vi "即时帮助.vi"() -> ()   [LabVIEW 2020]
panel:
  in  "确认":bool
  out "帮助信息":T1
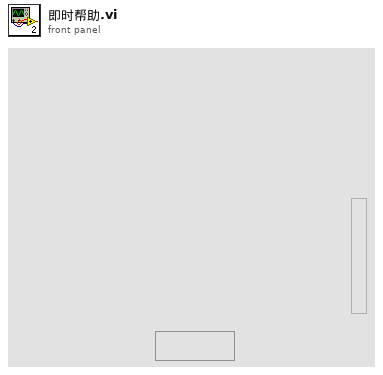
[diagram p1: front panel]
types:
  T1 = cluster{"名称":string, "图片":picture, "关键字":string, "程序文本":string}
  T2 = cluster{"名称":string, "关键字":string, "程序文本":string}
  T3 = typedef "imagedata.ctl" = cluster{"image type":i32, "image depth":i32, "image":u8[], "mask":u8[], "colors":u32[], "Rectangle":cluster{"left":i16, "top":i16, "right":i16, "bottom":i16}}
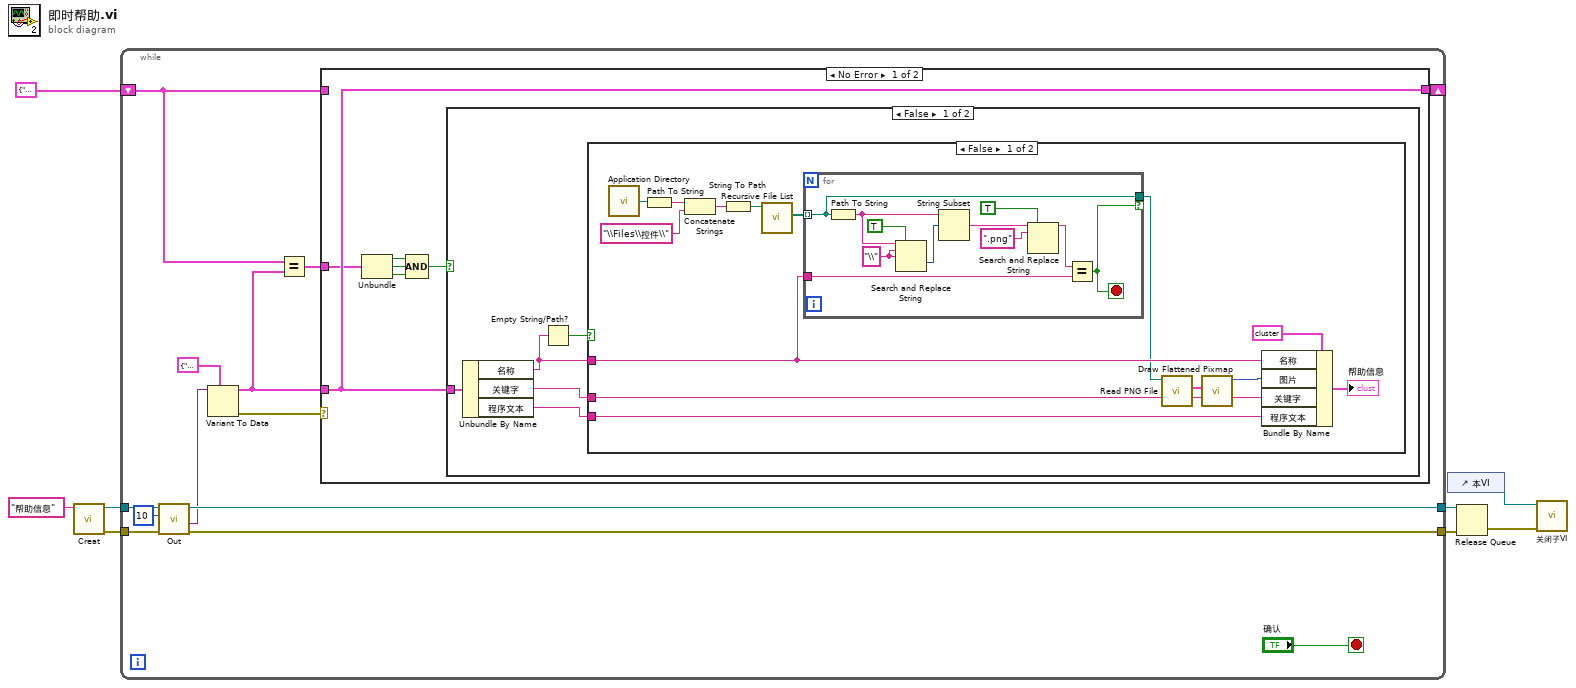
[diagram p0: block diagram]
diagram:
  n1 = call "Creat.vi"("名称"="帮助信息") -> ("错误输出"=w6:errorcluster, "队列输出"=w7:refnum<queue>)  [unwired: 9 in]
  n2 = while {
    tunnel: w7 -> [w21]
    tunnel: w6 -> [w20]
    shift-right: [w11] -> _
    shift-left: T2 {"名称"="", "关键字"="", "程序文本"=""} -> [w10]
    tunnel: [w19] -> w4
    tunnel: [w18] -> w5
    stop <- "确认" stop-if-true
    n3 = call "Out.vi"("错误输入"=w20, "超时毫秒(-1)"=10, "队列"=w21) -> ("错误输出"=w18:errorcluster, "数据"=w15:variant, "队列输出"=w19:refnum<queue>)  [unwired: 5 in, 1 out]
    n4 = Variant To Data(type=T2 {"名称"="", "关键字"="", "程序文本"=""}, Variant=w15) -> (data=w9:T2, error out=w12:errorcluster)  [unwired: 1 in]
    n5 = Equal?(x=w10, y=w9) -> (x = y?=w14:cluster{"名称":bool, "关键字":bool, "程序文本":bool})
    n6 = case shown="No Error" w12 {
      tunnel: w9 -> [w27 _]
      tunnel: w14 -> [w26 _]
      tunnel: [w27 w58] -> w11
      tunnel: w10 -> [_ w58]
      frame No Error {
        n7 = Unbundle(w26) -> ("名称"=w25:bool, "关键字"=w24:bool, "程序文本"=w23:bool)
        n8 = Compound Arithmetic op=AND(w25, w24, w23) -> (w22:bool)
        n9 = case shown="False" w22 {
          tunnel: w27 -> [w32 _]
          frame False {
            n10 = Unbundle By Name(w32) -> ("名称"=w29:string, "关键字"=w31:string, "程序文本"=w30:string)
            n11 = Empty String/Path?(string/path=w29) -> (empty?=w28:bool)
            n12 = case shown="False" w28 {
              tunnel: w31 -> [w45 _]
              tunnel: w30 -> [w44 _]
              tunnel: w29 -> [w34 _]
              frame False {
                n13 = call <vilib>:"Application Directory.vi"() -> ("Application Directory"=w40:path)
                n14 = Path To String(path=w40) -> (string=w39:string)
                n15 = Concatenate Strings(w39, "\\Files\\控件\\" ("名称或相对路径")) -> (w37:string)
                n16 = String To Path(string=w37) -> (path=w36:path)
                n17 = call <vilib>:"Recursive File List.vi"("Folder Path"=w36) -> ("All Files in Dir"=w35:path[])  [unwired: 6 in, 4 out]
                n18 = for {
                  tunnel: w35 -> [w50] mode=indexing
                  tunnel: [w50] -> w33 if=w47
                  tunnel: w34 -> [w48]
                  stop <- w47 stop-if-true
                  w56 = "\\" ("搜索字符串")
                  n19 = Path To String(path=w50) -> (string=w55:string)
                  n20 = Search and Replace String(replace all?=TRUE ("替换全部？(F)"), input string=w55, search string=w56, replace string=w56) -> (offset past replacement=w54:i32)  [unwired: 4 in, 3 out]
                  n21 = String Subset(string=w55, offset (0)=w54) -> (substring=w52:string)  [unwired: 1 in]
                  n22 = Search and Replace String(replace all?=TRUE ("替换全部？(F)"), input string=w52, search string=".png" ("搜索字符串")) -> (result string=w49:string)  [unwired: 5 in, 3 out]
                  n23 = Equal?(x=w49, y=w48) -> (x = y?=w47:bool)
                }
                n24 = call <vilib>:"Read PNG File.vi"("path to PNG file"=w33) -> ("image data"=w43:T3)  [unwired: 8 in, 2 out]
                n25 = call <vilib>:"Draw Flattened Pixmap.vi"("image data"=w43) -> ("new picture"=w42:picture)  [unwired: 8 in]
                n26 = Bundle By Name(cluster=T1 {"名称"="", "图片"=bytes[0], "关键字"="", "程序文本"=""} ("帮助信息"), "名称"=w34, "图片"=w42, "关键字"=w45, "程序文本"=w44) -> (→"帮助信息":T1)
              }
              frame True {
              }
            }
          }
          frame True {
          }
        }
      }
      frame Error {
      }
    }
  }
  n27 = control-ref of="本VI"() -> (w2:refnum<vi>)
  n28 = Release Queue(queue=w4, error in (no error)=w5) -> (error out=w1:errorcluster)  [unwired: 1 in, 2 out]
  n29 = call "关闭子VI.vi"("错误输入"=w1, "引用"=w2) -> ()  [unwired: 8 in, 2 out]
